vi "KE6221 -- PDelta Mode Set Params.vi"(0 "6221 Resource In":refnum<visa-resource-name>, 1 "Check For SCPI Errors? (T)":bool=TRUE, 7 "Pulsed Delta Mode Params In":T1={"High Level (A)"=0.001, "Low Level (A)"=0.0, "Pulse Width (s)"=0.00011, "Source Delay (s)"=1.6e-05, "Num Cycles Mode"=enum."Finite Count", "Finite Count"=1, "Ranging Mode"=enum."Best", "Num Low Meas Per Cycle"=enum."1", "Pulse Period (Num PLCs)"=5, "Pulse Sweep Mode Enabled?"=FALSE} {"Pulse Period (Num PLCs)" min=5 max=999990; "Source Delay (s)" min=1.6e-05 max=0.011966 format="%.3p"; "Pulse Width (s)" min=5e-05 max=0.012 format="%.3p"; "Finite Count" min=2 max=65536; "Low Level (A)" min=-0.105 max=0.0 format="%.3p"; "High Level (A)" min=0.0 max=0.105 format="%.3p"}, 11 "error in (no error)":errorcluster, 12 "Read Back Set Values? (T)":bool=TRUE) -> (4 "6221 Resource Out (dupl)":refnum<visa-resource-name>, 8 "Pulsed Delta Mode Params Out":T1={"High Level (A)"=0.001, "Low Level (A)"=0.0, "Pulse Width (s)"=0.00011, "Source Delay (s)"=1.6e-05, "Num Cycles Mode"=enum."Finite Count", "Finite Count"=1, "Ranging Mode"=enum."Best", "Num Low Meas Per Cycle"=enum."1", "Pulse Period (Num PLCs)"=5, "Pulse Sweep Mode Enabled?"=FALSE} {"Pulse Period (Num PLCs)" min=5 max=999990; "Source Delay (s)" min=1.6e-05 max=0.011966 format="%.3p"; "Pulse Width (s)" min=5e-05 max=0.012 format="%.3p"; "Finite Count" min=1 max=65536; "Low Level (A)" min=-0.105 max=0.0 format="%.3p"; "High Level (A)" min=0.0 max=0.105 format="%.3p"}, 15 "error out":errorcluster)   [LabVIEW 2019, in "Keithley 622x.lvlib"]
doc: "Sets the parameters for 'Pulsed Delta' measurements. Note that 'Pulsed Delta' measurements are only available on the 6221, and performing this measurement implies that the 6221 is being used in conjuction with a 2182/2182A nano-voltmeter."
uses:
  Keithley 622x.lvlib
  Typedefs/KE6221 -- PDelta Mode Params.ctl
  Low Level/Typedefs/KE622x -- Delta PDelta Mode High Level.ctl
  Low Level/Typedefs/KE622x -- Delta PDelta Mode Low Level.ctl
  Low Level/Typedefs/KE6221 -- PDelta Mode Pulse Width.ctl
  Low Level/Typedefs/KE6221 -- PDelta Mode Source Delay.ctl
  Low Level/Typedefs/KE622x -- Delta PDelta Mode Num Cycles Mode.ctl
  Low Level/Typedefs/KE622x -- Delta PDelta Mode Num Cycles.ctl
  Low Level/Typedefs/KE6221 -- PDelta Mode Ranging Mode.ctl
  Low Level/Typedefs/KE6221 -- PDelta Mode Num Low Meas.ctl
  Low Level/Typedefs/KE6221 -- PDelta Mode Pulse Period.ctl
  Trace Buf/Low Level/Typedefs/KE622x -- Trace Buf Size.ctl
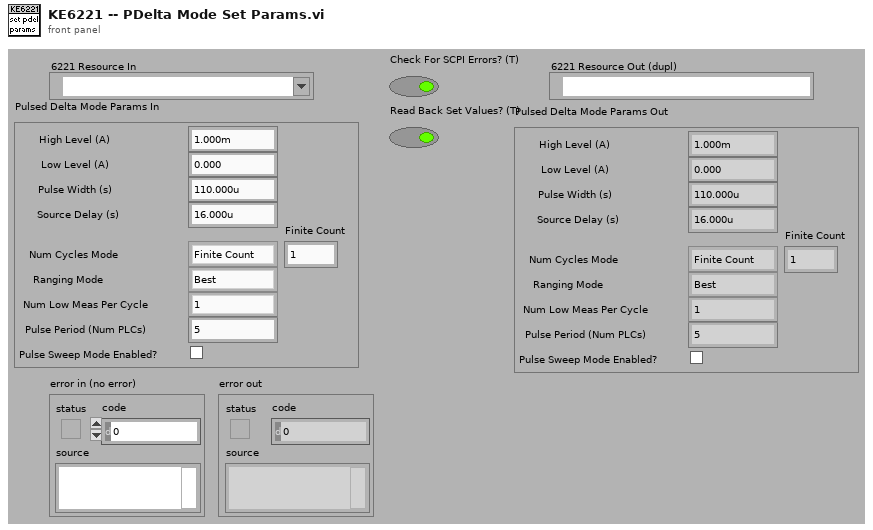
[diagram p1: front panel]
types:
  T1 = typedef "Keithley 622x.lvlib/KE6221 -- PDelta Mode Params.ctl" = cluster{"High Level (A)":T2, "Low Level (A)":T3, "Pulse Width (s)":T4, "Source Delay (s)":T5, "Num Cycles Mode":T6, "Finite Count":T7, "Ranging Mode":T8, "Num Low Meas Per Cycle":T9, "Pulse Period (Num PLCs)":T10, "Pulse Sweep Mode Enabled?":bool}
  T2 = typedef "Keithley 622x.lvlib/KE622x -- Delta PDelta Mode High Level.ctl" = dbl
  T3 = typedef "Keithley 622x.lvlib/KE622x -- Delta PDelta Mode Low Level.ctl" = dbl
  T4 = typedef "Keithley 622x.lvlib/KE6221 -- PDelta Mode Pulse Width.ctl" = dbl
  T5 = typedef "Keithley 622x.lvlib/KE6221 -- PDelta Mode Source Delay.ctl" = dbl
  T6 = typedef "Keithley 622x.lvlib/KE622x -- Delta PDelta Mode Num Cycles Mode.ctl" = enum16{"Finite Count", "Infinite"}
  T7 = typedef "Keithley 622x.lvlib/KE622x -- Delta PDelta Mode Num Cycles.ctl" = u32
  T8 = typedef "Keithley 622x.lvlib/KE6221 -- PDelta Mode Ranging Mode.ctl" = enum16{"Best", "Fixed"}
  T9 = typedef "Keithley 622x.lvlib/KE6221 -- PDelta Mode Num Low Meas.ctl" = enum16{"1", "2"}
  T10 = typedef "Keithley 622x.lvlib/KE6221 -- PDelta Mode Pulse Period.ctl" = u32
  T11 = typedef "Keithley 622x.lvlib/KE622x -- Trace Buf Size.ctl" = u32
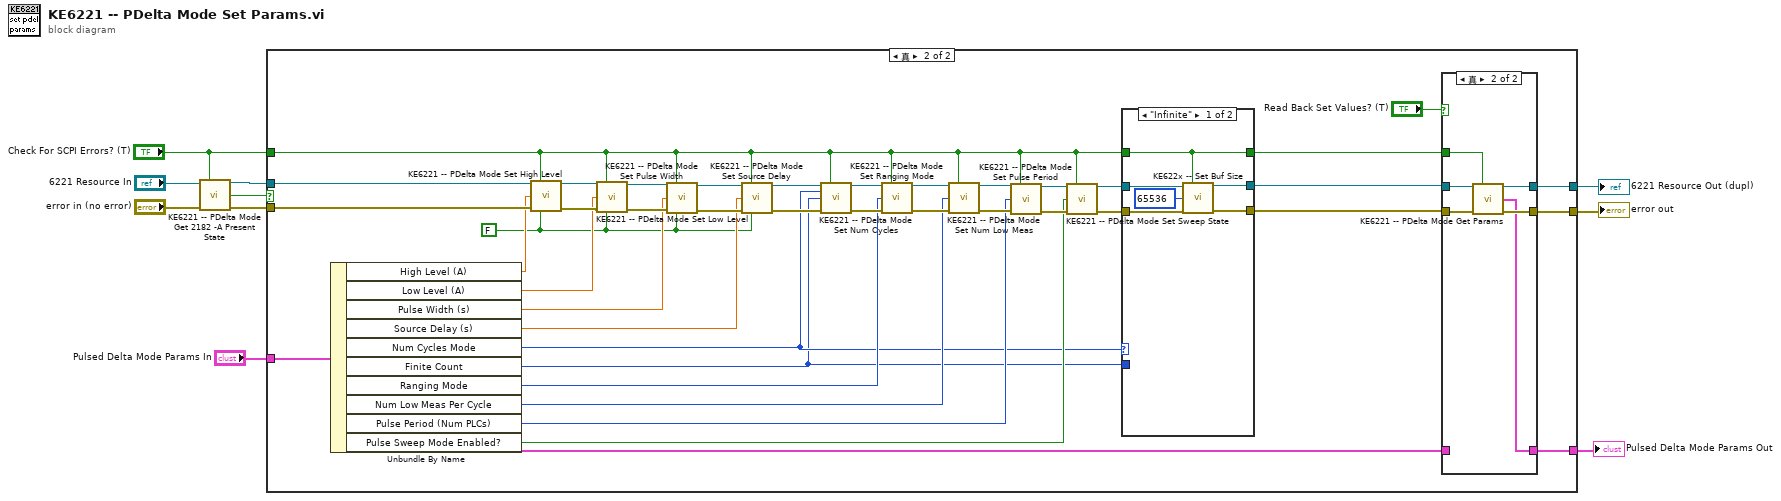
[diagram p0: block diagram]
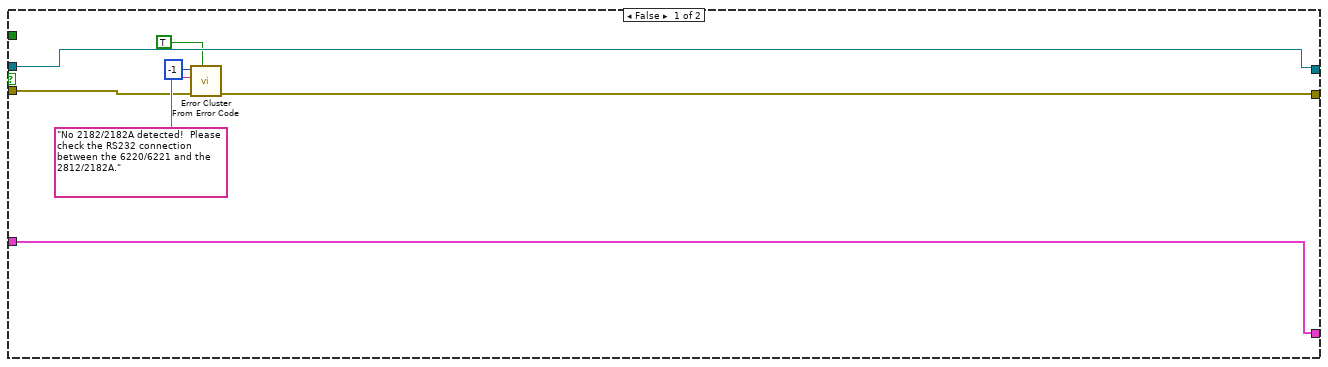
[diagram p2: hidden frame]
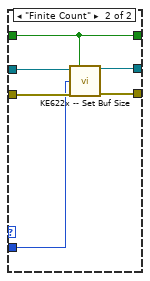
[diagram p3: hidden frame]
diagram:
  n1 = call "KE6221 -- PDelta Mode Get 2182 -A Present State.vi"("Resource In"="6221 Resource In", "Check For SCPI Errors? (T)"="Check For SCPI Errors? (T)", "error in (no error)"="error in (no error)") -> ("Resource Out (dupl)"=w6:refnum<visa-resource-name>, "2182/2182A Present?"=w4:bool, "error out"=w5:errorcluster)  [unwired: 10 in]
  n2 = case shown="真" w4 {
    tunnel: w6 -> [w14 w57]
    tunnel: w5 -> [w15 w56]
    tunnel: [w13 w30] -> w10
    tunnel: "Check For SCPI Errors? (T)" -> [_ w22]
    tunnel: [w12 w29] -> w9
    tunnel: [w14 w27] -> w8
    tunnel: "Pulsed Delta Mode Params In" -> [w12 w26]
    frame False {
      n3 = call <vilib>:"Error Cluster From Error Code.vi"("show call chain? (False)"=TRUE, "error in (no error)"=w15, "error message (\"\")"="No 2182/2182A detected!  Please check the RS232 connection between the 6220/6221 and the 2812/2182A.", "error code (0)"=-1) -> ("error out"=w13:errorcluster)  [unwired: 5 in]
    }
    frame True {
      w28 = FALSE ("Read Back Set Value? (T)")
      n4 = Unbundle By Name(w26) -> ("High Level (A)"=w39:T2, "Low Level (A)"=w38:T3, "Pulse Width (s)"=w37:T4, "Source Delay (s)"=w36:T5, "Num Cycles Mode"=w25:T6, "Finite Count"=w21:T7, "Ranging Mode"=w35:T8, "Num Low Meas Per Cycle"=w34:T9, "Pulse Period (Num PLCs)"=w33:T10, "Pulse Sweep Mode Enabled?"=w32:bool)
      n5 = call "KE6221 -- PDelta Mode Set High Level.vi"("Resource In"=w57, "Check For SCPI Errors? (T)"=w22, "High Level In (A)"=w39, "error in (no error)"=w56, "Read Back Set Value? (T)"=w28) -> ("Resource Out (dupl)"=w55:refnum<visa-resource-name>, "error out"=w54:errorcluster)  [unwired: 8 in, 1 out]
      n6 = call "KE6221 -- PDelta Mode Set Low Level.vi"("Resource In"=w55, "Check For SCPI Errors? (T)"=w22, "Low Level In (A)"=w38, "error in (no error)"=w54, "Read Back Set Value? (T)"=w28) -> ("Resource Out (dupl)"=w53:refnum<visa-resource-name>, "error out"=w52:errorcluster)  [unwired: 8 in, 1 out]
      n7 = call "KE6221 -- PDelta Mode Set Pulse Width.vi"("Resource In"=w53, "Check For SCPI Errors? (T)"=w22, "Pulse Width In (s)"=w37, "error in (no error)"=w52, "Read Back Set Value? (T)"=w28) -> ("Resource Out (dupl)"=w51:refnum<visa-resource-name>, "error out"=w50:errorcluster)  [unwired: 8 in, 1 out]
      n8 = call "KE6221 -- PDelta Mode Set Source Delay.vi"("Resource In"=w51, "Check For SCPI Errors? (T)"=w22, "Source Delay In (s)"=w36, "error in (no error)"=w50, "Read Back Set Value? (T)"=w28) -> ("Resource Out (dupl)"=w47:refnum<visa-resource-name>, "error out"=w46:errorcluster)  [unwired: 8 in, 1 out]
      n9 = call "KE6221 -- PDelta Mode Set Num Cycles.vi"("Resource In"=w47, "Check For SCPI Errors? (T)"=w22, "Num Cycles Mode"=w25, "Finite Count"=w21, "error in (no error)"=w46) -> ("Resource Out (dupl)"=w49:refnum<visa-resource-name>, "error out"=w48:errorcluster)  [unwired: 9 in]
      n10 = call "KE6221 -- PDelta Mode Set Ranging Mode.vi"("Resource In"=w49, "Check For SCPI Errors? (T)"=w22, "Ranging Mode"=w35, "error in (no error)"=w48) -> ("Resource Out (dupl)"=w43:refnum<visa-resource-name>, "error out"=w42:errorcluster)  [unwired: 10 in]
      n11 = call "KE6221 -- PDelta Mode Set Num Low Meas.vi"("Resource In"=w43, "Check For SCPI Errors? (T)"=w22, "Num Low Meas Per Cycle"=w34, "error in (no error)"=w42) -> ("Resource Out (dupl)"=w41:refnum<visa-resource-name>, "error out"=w40:errorcluster)  [unwired: 10 in]
      n12 = call "KE6221 -- PDelta Mode Set Pulse Period.vi"("Resource In"=w41, "Check For SCPI Errors? (T)"=w22, "Pulse Period (Num PLCs)"=w33, "error in (no error)"=w40) -> ("Resource Out (dupl)"=w45:refnum<visa-resource-name>, "error out"=w44:errorcluster)  [unwired: 10 in]
      n13 = call "KE6221 -- PDelta Mode Set Sweep State.vi"("Resource In"=w45, "Check For SCPI Errors? (T)"=w22, "Enable Sweep?"=w32, "error in (no error)"=w44) -> ("Resource Out (dupl)"=w24:refnum<visa-resource-name>, "error out"=w23:errorcluster)  [unwired: 10 in]
      n14 = case shown="\"Infinite\"" w25 {
        tunnel: w24 -> [w63 w69]
        tunnel: w23 -> [w61 w68]
        tunnel: w22 -> [w60 w64]
        tunnel: w21 -> [_ w67]
        tunnel: [w58 w66] -> w19
        tunnel: [w59 w65] -> w20
        tunnel: [w60 w64] -> w18
        frame "Infinite" {
          n15 = call "KE622x -- Set Buf Size.vi"("Resource In"=w63, "Check For SCPI Errors? (T)"=w60, "Buffer Size (Num Readings)"=T11 65536, "error in (no error)"=w61) -> ("Resource Out (dupl)"=w59:refnum<visa-resource-name>, "error out"=w58:errorcluster)  [unwired: 10 in]
        }
        frame "Finite Count" {
          n16 = call "KE622x -- Set Buf Size.vi"("Resource In"=w69, "Check For SCPI Errors? (T)"=w64, "Buffer Size (Num Readings)"=w67, "error in (no error)"=w68) -> ("Resource Out (dupl)"=w65:refnum<visa-resource-name>, "error out"=w66:errorcluster)  [unwired: 10 in]
        }
      }
      n17 = case shown="真" "Read Back Set Values? (T)" {
        tunnel: w20 -> [w72 w78]
        tunnel: w19 -> [w71 w77]
        tunnel: [w72 w76] -> w27
        tunnel: [w71 w75] -> w30
        tunnel: w18 -> [_ w74]
        tunnel: w26 -> [w70 _]
        tunnel: [w70 w73] -> w29
        frame False {
        }
        frame True {
          n18 = call "KE6221 -- PDelta Mode Get Params.vi"("6221 Resource In"=w78, "Check For SCPI Errors? (T)"=w74, "error in (no error)"=w77) -> ("6221 Resource Out (dupl)"=w76:refnum<visa-resource-name>, "Pulsed Delta Mode Params"=w73:T1, "error out"=w75:errorcluster)  [unwired: 10 in]
        }
      }
    }
  }
  "error out" <- w10
  "Pulsed Delta Mode Params Out" <- w9
  "6221 Resource Out (dupl)" <- w8
